vi "Do This.vi"(8 "error in (no error)":errorcluster, 10 "Status Events":refnum<class "Status Events.lvclass">, 11 "Run UTF in":refnum<class "Run UTF.lvclass">) -> (0 "error out":errorcluster, 3 "Run UTF out":refnum<class "Run UTF.lvclass">)   [LabVIEW 2014, in "Run UTF.lvclass"]
uses:
  Run UTF.lvclass
  Shared/Classes/Status Events/Status Events.lvclass
  Run UTF.lvclass/Run UTF.ctl
  Classes/Job/Job.lvclass/Job.ctl
  <vilib>/NI/UTF Junit Report/utf junit report.lvlib
  Classes/Job/Job.lvclass
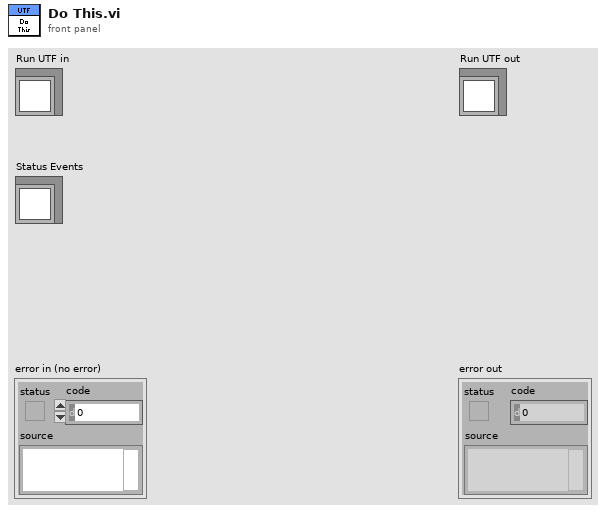
[diagram p1: front panel]
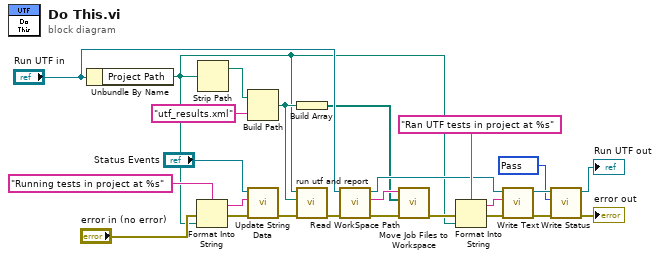
[diagram p0: block diagram]
diagram:
  w21 = u16 200 items=["Service Error"=504, "Abort"=503, "Fail"=500, "Pass"=200] ("Status")
  n1 = Unbundle By Name("Run UTF in") -> ("Project Path"=w2:path)
  n2 = Format Into String(format string="Running tests in project at %s", error in="error in (no error)", w2) -> (resulting string=w12:string, error out=w14:errorcluster)  [unwired: 1 in]
  n3 = Strip Path(path=w2) -> (stripped path=w1:path)  [unwired: 1 out]
  n4 = Build Path(base path=w1, name or relative path="utf_results.xml") -> (appended path=w3:path)
  n5 = call "Update String Data.vi"("error in (no error)"=w14, "String Data"=w12, "Status Updater in"="Status Events") -> ("error out"=w10:errorcluster)  [unwired: 7 in, 1 out]
  n6 = Build Array(w3) -> (w6:path[])
  n7 = call <vilib>:"run utf and report.vi"("error in (no error)"=w10, "junit report file path"=w3, "project file path"=w2) -> ("Error Out"=w5:errorcluster)  [unwired: 8 in]
  n8 = call "Read WorkSpace Path.vi"("error in (no error)"=w5, "Job in"="Run UTF in") -> ("error out"=w7:errorcluster, "WorkSpace Path"=w9:string, "Job out"=w8:refnum<class "Run UTF.lvclass">)  [unwired: 7 in]
  n9 = call "Move Job Files to Workspace.vi"("error in (no error)"=w7, "Generated Files"=w6, "Workspace Path"=w9) -> ("error out"=w4:errorcluster)  [unwired: 8 in]
  n10 = Format Into String(format string="Ran UTF tests in project at %s", error in=w4, w2) -> (resulting string=w20:string, error out=w19:errorcluster)  [unwired: 1 in]
  n11 = call "Write Text.vi"("error in (no error)"=w19, "Text"=w20, "Job in"=w8) -> ("error out"=w22:errorcluster, "Job out"=w25:refnum<class "Run UTF.lvclass">)  [unwired: 7 in]
  n12 = call "Write Status.vi"("error in (no error)"=w22, "Status"=w21, "Job in"=w25) -> ("error out"=→"error out":errorcluster, "Job out"=→"Run UTF out":refnum<class "Run UTF.lvclass">)  [unwired: 7 in]
